vi "SCC Not A Source Control Reference.vi"(8 "error in (no error)":errorcluster, 10 "source control reference in":T1) -> (0 "error out":errorcluster, 2 "not a source control reference?":bool)   [LabVIEW 2017, in "NI_SCC.lvlib"]
doc: "Specifies whether a source control reference is a valid refnum."
uses:
  <vilib>/SourceControl/sccapi/NI_SCC.lvlib
  <vilib>/SourceControl/sccapi/SCCAPI Refnum.ctl
  <vilib>/SourceControl/sccapi/SCCAPI SCC Operations.ctl
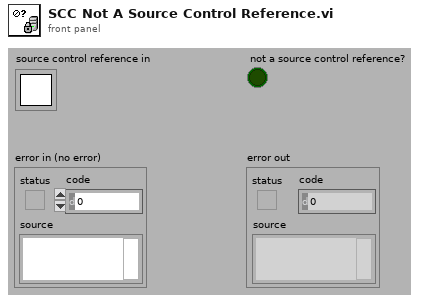
[diagram p1: front panel]
types:
  T1 = typedef "NI_SCC.lvlib/SCCAPI Refnum.ctl" = refnum<k1>
  T2 = typedef "NI_SCC.lvlib/SCCAPI SCC Operations.ctl" = enum16{"Add", "Check In", "Check Out", "Close Project", "Compare Files", "Compare VIs", "Configure Project", "File History", "File Properties", "File Status", "Find All Providers", "Get Advanced Command Options", "Get File Copy", "Get Latest Version", "Get Project Name", "Get StaticVI Path", "Initialize", "Not A Source Control Reference", "Open Project", "Provider Supports Functionality", "Remove", "Run Provider", "Undo Check Out", "Uninitialize", "Is File In Local Path"}
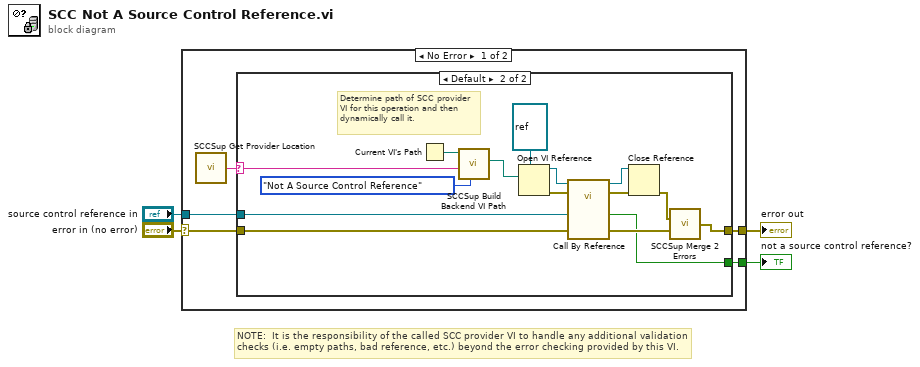
[diagram p0: block diagram]
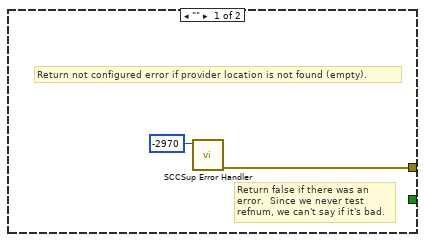
[diagram p2: hidden frame]
diagram:
  # "NOTE:  It is the responsibility of the called SCC provider VI to handle any additional validation checks (i.e. empty paths, bad reference, etc.) beyond the error checking provided by this VI."
  n1 = case shown="No Error" "error in (no error)" {
    selector: "error in (no error)" -> [w6 w27]
    tunnel: [w9 w27] -> w4
    tunnel: [w8 _] -> w3
    tunnel: "source control reference in" -> [w7 _]
    frame No Error {
      n2 = call <vilib>:"SCCSup Get Provider Location.vi"() -> ("provider location"=w5:string)  [unwired: 6 in]
      n3 = case shown="Default" w5 {
        selector: w5 -> [_ w13]
        tunnel: [w10 w16] -> w9
        tunnel: [_ w15] -> w8
        tunnel: w7 -> [_ w14]
        tunnel: w6 -> [_ w12]
        frame "" {
          # "Return false if there was an error.  Since we never test refnum, we can't say if it's bad."
          # "Return not configured error if provider location is not found (empty)."
          n4 = call <vilib>:"SCCSup Error Handler.vi"("scc error code"=-2970 ("code")) -> ("error out"=w10:errorcluster)  [unwired: 10 in]
        }
        frame Default {
          # "Determine path of SCC provider VI for this operation and then dynamically call it."
          n5 = Current VI's Path() -> (path=w20:path)
          n6 = call <vilib>:"SCCSup Build Backend VI Path.vi"("scc operation"=SCCAPI_SCC_Operations."Not A Source Control Reference", "provider location"=w13, "caller path"=w20) -> ("scc backend VI path"=w19:path)  [unwired: 8 in]
          n7 = Open VI Reference(type specifier VI Refnum (for type only)=refnum<vi> refnum, vi path=w19) -> (vi reference=w17:refnum<vi>, error out=w25:errorcluster)  [unwired: 4 in]
          n8 = call-by-ref "?"(reference=w17, error in=w25, "error in (no error)"=w12, "source control reference in"=w14) -> (reference out=w24:refnum<vi>, error out=w23:errorcluster, 0:"error out"=w21:errorcluster, "not an SCC refnum"=w15:bool)  [unwired: 8 in]
          n9 = Close Reference(reference=w24, error in (no error)=w23) -> (error out=w22:errorcluster)
          n10 = call <vilib>:"SCCSup Merge 2 Errors.vi"("Error IO 1"=w22, "Error IO 2"=w21) -> ("Error IO out"=w16:errorcluster)  [unwired: 13 in]
        }
      }
    }
    frame Error {
      # "Return false if there was an error.  Since we never test refnum, we can't say if it's bad."
    }
  }
  "not a source control reference?" <- w3
  "error out" <- w4
